vi "GETSECONDBALL.vi"   [LabVIEW 2016, in "Test2.lvrbt"]
uses:
  Test2.lvrbt
  <vilib>/NXT/Block Support/NXT_InputPort.ctl
  <vilib>/NXT/Hardware/Plugins/Tetrix DC Motor/TetrixDCMotorAddress.ctl
  <vilib>/NXT/Hardware/Plugins/Tetrix 180 deg Servo/Tetrix180ServoAddress.ctl
  <vilib>/NXT/NXTIO Xnodes/NXTIONodeSubVIs/TETRIX IO Move Servos.vi
  <vilib>/NXT/Dual Mode Library/Waits/Wait_Num.vi
  <vilib>/NXT/NXTIO Xnodes/NXTIONodeSubVIs/TETRIX IO Move DC Motors.vi
  <vilib>/NXT/Dual Mode Library/Waits/Wait_EV3_Ultrasonic_Centimeters_Further.vi
  <vilib>/NXT/NXTIO Xnodes/NXTIONodeSubVIs/TETRIX IO Stop DC Motors.vi
  <vilib>/NXT/Dual Mode Library/Waits/Wait_EV3_Ultrasonic_Centimeter_Closer.vi
  <vilib>/NXT/NXTIO Xnodes/AddressXNode/NXTIOAddress.xnode
  <vilib>/NXT/Subs/LVHSConnector.ctl
  <vilib>/NXT/NXTIO Xnodes/NXTIOXNode/NXTIO.xnode
  <vilib>/NXT/LegoClasses/BrickReference/BrickReference.lvclass
types:
  T1 = typedef "NXT_InputPort.ctl" = u32
  T2 = typedef "Tetrix180ServoAddress.ctl" = i32
  T3 = cluster{"Tetrix180Servo":T2, "Tetrix180Servo":T2, "Tetrix180Servo":T2, "Tetrix180Servo":T2, "Tetrix180Servo":T2, "Tetrix180Servo":T2}
  T4 = typedef "TetrixDCMotorAddress.ctl" = i32
  T5 = typedef "LVHSConnector.ctl" = refnum<class "BrickReference.lvclass">
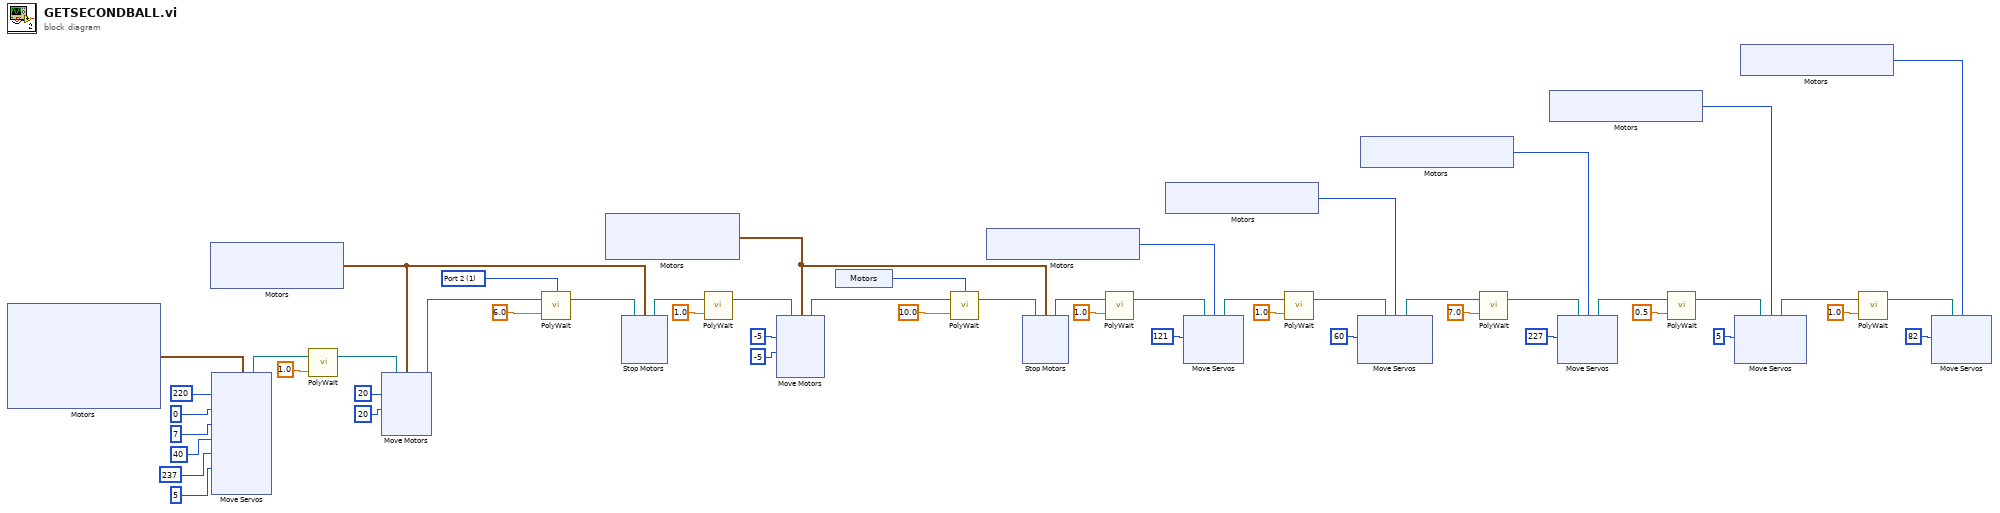
[diagram p0: block diagram]
diagram:
  w48 = T1 1 items=["Port 1", "Port 2", "Port 3", "Port 4"] ("Port (Port 1)")
  n1 = xnode "Motors"() -> ("Motor"=w43:T3)
  n2 = xnode "Motors"() -> ("Motor"=w44:cluster{"TetrixDCMotor":T4, "TetrixDCMotor":T4})
  n3 = xnode "Move Servos"("Position 6"=u8 5, "Position 5"=u8 237, "Position 4"=u8 40, "Position 3"=u8 7, "Position 2"=u8 0, "Position 1"=u8 220, "Motors"=w43) -> ("NXT/EV3"=w36:T5)  [unwired: 1 in]
  n4 = call-poly <vilib>:"PolyWait.vi"("Time (1 sec)"=sgl 1.0, "NXT/EV3"=w36) -> ("NXT/EV3"=w45:T5)  [unwired: 2 in]
  n5 = xnode "Move Motors"("Power/Speed 2"=i8 20, "Power/Speed 1"=i8 20, "Motors"=w44, "NXT/EV3"=w45) -> ("NXT/EV3"=w51:T5)
  n6 = call-poly <vilib>:"PolyWait.vi"("Centimeters (50)"=sgl 6.0, "NXT/EV3"=w51, "Port (Port 1)"=w48) -> ("NXT/EV3"=w49:T5)  [unwired: 1 in]
  n7 = xnode "Motors"() -> ("Motor"=w31:cluster{"TetrixDCMotor":T4, "TetrixDCMotor":T4})
  n8 = xnode "Stop Motors"("Motors"=w44, "NXT/EV3"=w49) -> ("NXT/EV3"=w35:T5)
  n9 = call-poly <vilib>:"PolyWait.vi"("Time (1 sec)"=sgl 1.0, "NXT/EV3"=w35) -> ("NXT/EV3"=w26:T5)  [unwired: 2 in]
  n10 = xnode "Move Motors"("Power/Speed 2"=i8 -5, "Power/Speed 1"=i8 -5, "Motors"=w31, "NXT/EV3"=w26) -> ("NXT/EV3"=w33:T5)
  n11 = xnode "Motors"() -> ("Sensor"=w28:T1)
  n12 = call-poly <vilib>:"PolyWait.vi"("Centimeters (40)"=sgl 10.0 ("Centimeters (50)"), "NXT/EV3"=w33, "Port (Port 1)"=w28) -> ("NXT/EV3"=w32:T5)  [unwired: 1 in]
  n13 = xnode "Motors"() -> ("Motor"=w5:T2)
  n14 = xnode "Stop Motors"("Motors"=w31, "NXT/EV3"=w32) -> ("NXT/EV3"=w1:T5)
  n15 = call-poly <vilib>:"PolyWait.vi"("Time (1 sec)"=sgl 1.0, "NXT/EV3"=w1) -> ("NXT/EV3"=w2:T5)  [unwired: 2 in]
  n16 = xnode "Motors"() -> ("Motor"=w25:T2)
  n17 = xnode "Move Servos"("Position 1"=u8 121, "Motors"=w5, "NXT/EV3"=w2) -> ("NXT/EV3"=w3:T5)
  n18 = call-poly <vilib>:"PolyWait.vi"("Time (1 sec)"=sgl 1.0, "NXT/EV3"=w3) -> ("NXT/EV3"=w7:T5)  [unwired: 2 in]
  n19 = xnode "Move Servos"("Position 1"=u8 60, "Motors"=w25, "NXT/EV3"=w7) -> ("NXT/EV3"=w22:T5)
  n20 = xnode "Motors"() -> ("Motor"=w21:T2)
  n21 = call-poly <vilib>:"PolyWait.vi"("Time (1 sec)"=sgl 7.0, "NXT/EV3"=w22) -> ("NXT/EV3"=w19:T5)  [unwired: 2 in]
  n22 = xnode "Motors"() -> ("Motor"=w16:T2)
  n23 = xnode "Move Servos"("Position 1"=u8 227, "Motors"=w21, "NXT/EV3"=w19) -> ("NXT/EV3"=w17:T5)
  n24 = call-poly <vilib>:"PolyWait.vi"("Time (1 sec)"=sgl 0.5, "NXT/EV3"=w17) -> ("NXT/EV3"=w14:T5)  [unwired: 2 in]
  n25 = xnode "Move Servos"("Position 1"=u8 5, "Motors"=w16, "NXT/EV3"=w14) -> ("NXT/EV3"=w12:T5)
  n26 = xnode "Motors"() -> ("Motor"=w10:T2)
  n27 = call-poly <vilib>:"PolyWait.vi"("Time (1 sec)"=sgl 1.0, "NXT/EV3"=w12) -> ("NXT/EV3"=w9:T5)  [unwired: 2 in]
  n28 = xnode "Move Servos"("Position 1"=u8 82, "Motors"=w10, "NXT/EV3"=w9) -> ()  [unwired: 1 out]
